vi "CreateFunctions.vi"(7 "PythonConverter_BD in":refnum<class "PyConvBD.lvclass">, 8 "error in":errorcluster, 11 "Diagram in":refnum<class "Diagram.lvclass">) -> (0 "error out":errorcluster, 3 "Diagram out":refnum<class "Diagram.lvclass">, 4 "create functions":string, 5 "PythonConverter_BD out":refnum<class "PyConvBD.lvclass">)   [LabVIEW 2014, in "Raspberry Pi Compatible Compiler for LabVIEW.lvlib" / "Diagram.lvclass"]
uses:
  Diagram.lvclass
  Python/PythonConverter_BD/PyConvBD.lvclass
  Diagram.lvclass/Diagram.ctl
  Python/Parsing/ClassTypeTD.ctl
  GrowableFunction/GrowableFunction.lvclass
  Function/Function.lvclass
  SubVI/SubVI.lvclass
  Python/Parsing/Python Functions.lvlib
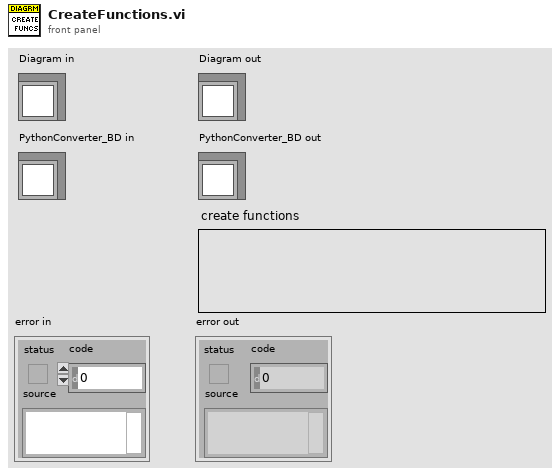
[diagram p1: front panel]
types:
  T1 = typedef "Raspberry Pi Compatible Compiler for LabVIEW.lvlib/Python Functions.lvlib/ClassTypeTD.ctl" = enum16{"class", "function"}
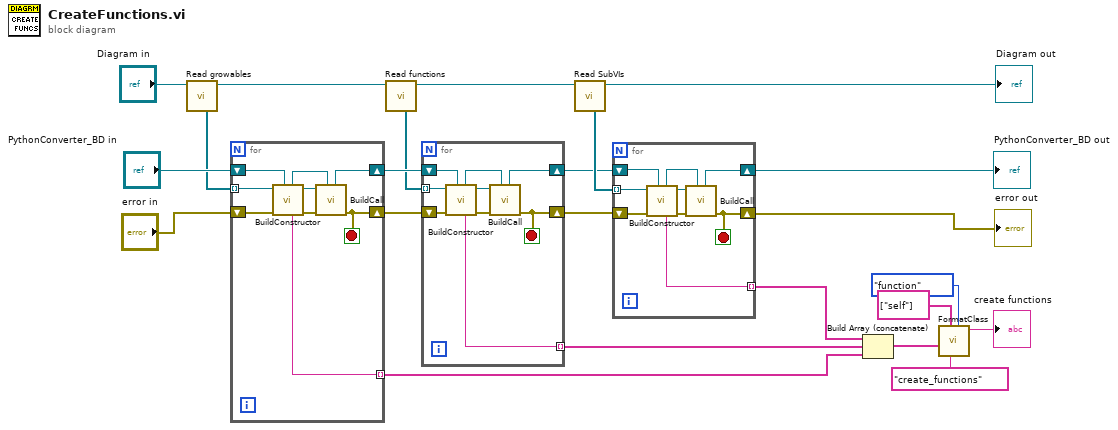
[diagram p0: block diagram]
diagram:
  n1 = call "Read growables.vi"("Diagram in"="Diagram in") -> ("Diagram out"=w3:refnum<class "Diagram.lvclass">, "growables"=w2:refnum<class "GrowableFunction.lvclass">[])  [unwired: 7 in]
  n2 = for {
    tunnel: w2 -> [w31] mode=indexing
    shift-right: [w27] -> w19
    shift-left: "PythonConverter_BD in" -> [w32]
    shift-right: [w28] -> w18
    shift-left: "error in" -> [w30]
    tunnel: [w26] -> w14 mode=indexing
    stop <- w28 stop-if-true
    n3 = call-dynamic "BuildConstructor.vi"("PythonConverter_BD in"=w32, "error in"=w30, "Function in"=w31) -> ("error out"=w29:errorcluster, "Function out"=w24:refnum<class "GrowableFunction.lvclass">, "constructor"=w26:string, "PythonConverter_BD out"=w25:refnum<class "PyConvBD.lvclass">)  [unwired: 5 in]
    n4 = call-dynamic "BuildCall.vi"("PythonConverter_BD in"=w25, "error in"=w29, "Function in"=w24) -> ("error out"=w28:errorcluster, "PythonConverter_BD out"=w27:refnum<class "PyConvBD.lvclass">)  [unwired: 6 in, 1 out]
  }
  n5 = call "Read functions.vi"("Diagram in"=w3) -> ("Diagram out"=w4:refnum<class "Diagram.lvclass">, "functions"=w5:refnum<class "Function.lvclass">[])  [unwired: 7 in]
  n6 = for {
    tunnel: w5 -> [w40] mode=indexing
    shift-right: [w33] -> w10
    shift-left: w19 -> [w41]
    shift-right: [w35] -> w9
    shift-left: w18 -> [w39]
    tunnel: [w38] -> w15 mode=indexing
    stop <- w35 stop-if-true
    n7 = call-dynamic "BuildConstructor.vi"("PythonConverter_BD in"=w41, "error in"=w39, "Function in"=w40) -> ("error out"=w37:errorcluster, "Function out"=w36:refnum<class "Function.lvclass">, "constructor"=w38:string, "PythonConverter_BD out"=w34:refnum<class "PyConvBD.lvclass">)  [unwired: 5 in]
    n8 = call-dynamic "BuildCall.vi"("PythonConverter_BD in"=w34, "error in"=w37, "Function in"=w36) -> ("error out"=w35:errorcluster, "PythonConverter_BD out"=w33:refnum<class "PyConvBD.lvclass">)  [unwired: 6 in, 1 out]
  }
  n9 = call "Read SubVIs.vi"("Diagram in"=w4) -> ("Diagram out"=→"Diagram out":refnum<class "Diagram.lvclass">, "SubVIs"=w11:refnum<class "SubVI.lvclass">[])  [unwired: 7 in]
  n10 = for {
    tunnel: w11 -> [w49] mode=indexing
    shift-right: [w45] -> w7
    shift-left: w10 -> [w50]
    shift-right: [w43] -> w8
    shift-left: w9 -> [w48]
    tunnel: [w47] -> w6 mode=indexing
    stop <- w43 stop-if-true
    n11 = call-dynamic "BuildConstructor.vi"("PythonConverter_BD in"=w50, "error in"=w48, "SubVI in"=w49) -> ("error out"=w46:errorcluster, "SubVI out"=w44:refnum<class "SubVI.lvclass">, "constructor"=w47:string, "PythonConverter_BD out"=w42:refnum<class "PyConvBD.lvclass">)  [unwired: 5 in]
    n12 = call-dynamic "BuildCall.vi"("PythonConverter_BD in"=w42, "error in"=w46, "SubVI in"=w44) -> ("error out"=w43:errorcluster, "PythonConverter_BD out"=w45:refnum<class "PyConvBD.lvclass">)  [unwired: 6 in, 1 out]
  }
  "error out" <- w8
  "PythonConverter_BD out" <- w7
  n13 = Build Array (concatenate)(w6, w15, w14) -> (w13:string[])
  n14 = call "FormatClass.vi"("type"=ClassTypeTD."function", "name"="create_functions" ("initial string"), "parameters/ancestors"=string[] ["self"], "body"=w13) -> ("python"=→"create functions":string)  [unwired: 7 in]
